vi "Update Status to Screen.vi"() -> (10 "output cluster":cluster{"Cluster":cluster{"Part ID":string}})   [LabVIEW 2021]
panel:
  out "error out":errorcluster
  out "Serial Number":dbl
  in  "error in":errorcluster
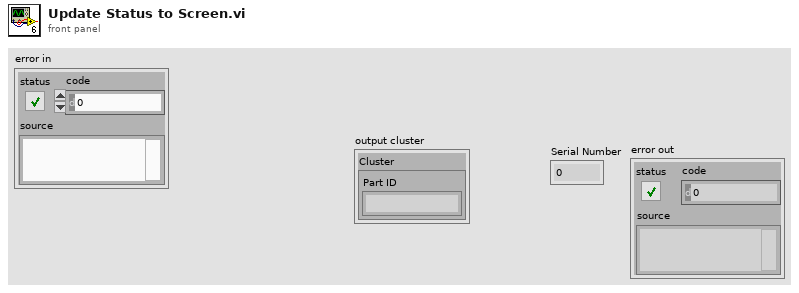
[diagram p1: front panel]
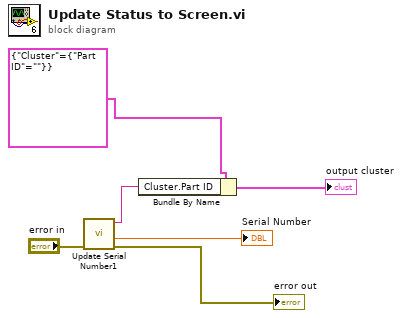
[diagram p0: block diagram]
diagram:
  n1 = call "Update Serial Number1.vi"("error in"="error in") -> ("error out"=→"error out":errorcluster, "Serial Number"=→"Serial Number":dbl, "Serial number"=w2:string)  [unwired: 8 in]
  n2 = Bundle By Name(cluster=cluster{"Cluster":cluster{"Part ID":string}} {"Cluster"={"Part ID"=""}}, "Cluster.Part ID"=w2) -> (→"output cluster":cluster{"Cluster":cluster{"Part ID":string}})
